vi "(SubVI)AOMvolt-Power Calibration for 1064-v2.vi"(6 "instrument handle":refnum<visa-resource-name>, 7 "error in (no error)":errorcluster {"code" format="%.0x"}) -> (0 "XY Graph":cluster{dbl[], dbl[]}[](graph), 1 "Raw data":T1, 3 "Choosed AOM volt":dbl, 4 "Choosed laser power (mW)":dbl format="%#_13g")   [LabVIEW 2014]
uses:
  <vilib>/Analysis/polynomials.llb/Scalar Polynomial Evaluation (DBL).vi
  <vilib>/Utility/file.llb/Write To Spreadsheet File (DBL).vi
  <vilib>/Analysis/NI_AALPro.lvlib
panel:
  out "Voltage for AOM":dbl
  out "powermeter readout (mW)":dbl
  in  "scan step #":dbl=20.0
  in  "Set laser power (mW)":dbl=10.0 format="%#_13g"
  in  "Scanning cycles":dbl=1.0
  in  "milliseconds to wait":u32=300
  out "voltage step size":dbl=0.25
  in  "Min voltage":dbl=0.1
  in  "Max voltage":dbl=5.0
  in  "save cal curve?":bool
  out "Fit AOM volt(V)":dbl[](array[numeric])
  out "Fit laser power (mW)":dbl[](array[numeric])
  out "Polynomial Coefficients":dbl[](array[numeric]) format="%0.2f"
  out "power":dbl
  out "current voltage":dbl
  in  "stop":bool
  # "continuous scaning power \nover AOM voltage range"
  # "**activate \ncontinuous power\ncontinuous AOM"
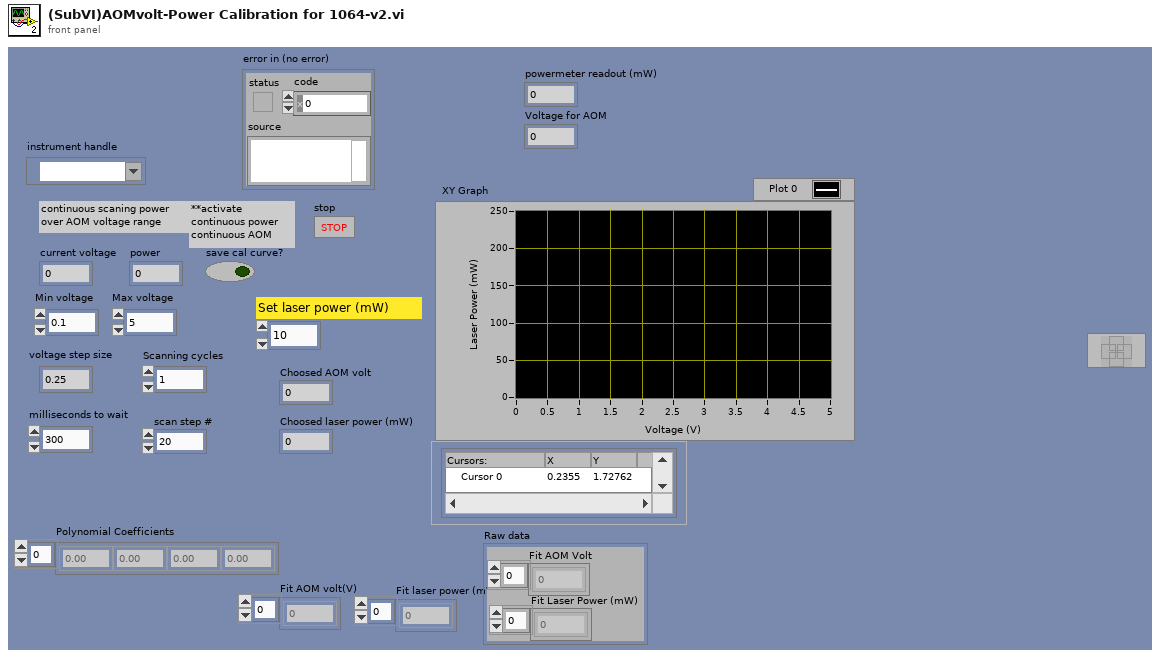
[diagram p1: front panel]
types:
  T1 = cluster{"Fit AOM Volt":dbl[], "Fit Laser Power (mW)":dbl[]}
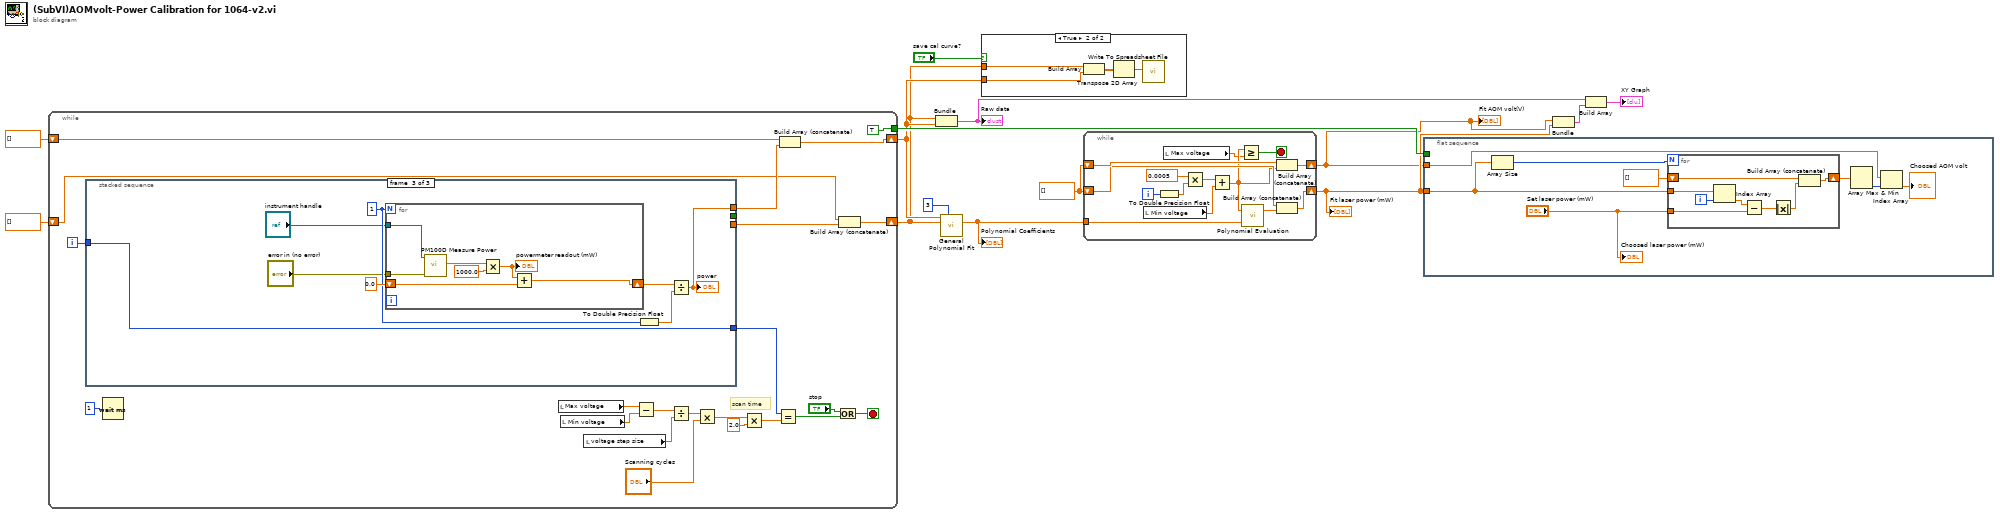
[diagram p0: block diagram]
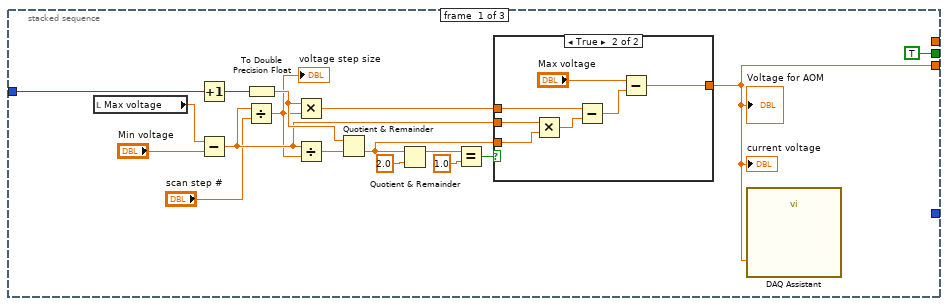
[diagram p3: hidden frame]
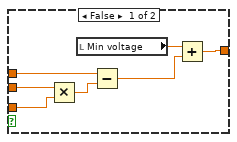
[diagram p4: hidden frame]
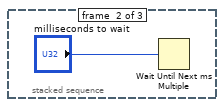
[diagram p5: hidden frame]
diagram:
  w10 = dbl[] []
  n1 = while {
    shift-right: [w34] -> w7
    shift-left: dbl[] [] -> [w31]
    shift-right: [w35] -> w6
    shift-left: dbl[] [] -> [w30]
    tunnel: [TRUE] -> w12
    i -> [w28]
    stop <- w26 stop-if-true
    # "scan time"
    n2 = stacked-sequence {
      tunnel: [w38 _ _] -> w33
      tunnel: [_ _ w72] -> w32
      tunnel: [TRUE _ _] -> _
      tunnel: w28 -> [w45 _ w75]
      tunnel: [_ _ w75] -> w25
      frame #0 {
        n3 = local read "Max voltage"() -> (w43:dbl)
        n4 = Increment(x=w45) -> (x+1=w52:i32)
        n5 = Subtract(x=w43, y="Min voltage") -> (x-y=w41:dbl)
        n6 = Divide(x=w41, y="scan step #") -> (x/y=w39:dbl)
        "voltage step size" <- w39
        n7 = To Double Precision Float(number=w52) -> (double precision float=w44:dbl)
        n8 = Multiply(x=w44, y=w39) -> (x*y=w51:dbl)
        n9 = Divide(x=w41, y=w39) -> (x/y=w42:dbl)
        n10 = Quotient & Remainder(x=w44, y=w42) -> (floor(x/y)=w46:dbl)  [unwired: 1 out]
        n11 = Quotient & Remainder(x=w46, y=2.0) -> (x-y*floor(x/y)=w48:dbl)  [unwired: 1 out]
        n12 = Equal?(x=w48, y=1.0) -> (x = y?=w49:bool)
        n13 = case shown="True" w49 {
          tunnel: w51 -> [w58 w66]
          tunnel: [w60 w67] -> w38
          tunnel: w46 -> [w59 w63]
          tunnel: w41 -> [w55 w61]
          frame False {
            n14 = Multiply(x=w55, y=w59) -> (x*y=w57:dbl)
            n15 = local read "Min voltage"() -> (w54:dbl)
            n16 = Subtract(x=w58, y=w57) -> (x-y=w56:dbl)
            n17 = Add(x=w54, y=w56) -> (x+y=w60:dbl)
          }
          frame True {
            n18 = Multiply(x=w61, y=w63) -> (x*y=w65:dbl)
            n19 = Subtract(x=w66, y=w65) -> (x-y=w64:dbl)
            n20 = Subtract(x="Max voltage", y=w64) -> (x-y=w67:dbl)
          }
        }
        "current voltage" <- w38
        "Voltage for AOM" <- w38
        n21 = call "DAQ Assistant"("data"=w38) -> ()  [unwired: 17 in, 2 out]
      }
      frame #1 {
        n22 = Wait Until Next ms Multiple(millisecond multiple="milliseconds to wait") -> ()  [unwired: 1 out]
      }
      frame #2 {
        w73 = 1
        n23 = for {
          N: w73 -> [_]
          shift-right: [w83] -> w74
          shift-left: 0.0 -> [w82]
          tunnel: "instrument handle" -> [w81]
          tunnel: "error in (no error)" -> [w80]
          n24 = call <instrlib>:"PM100D Measure Power.vi"("error in (no error)"=w80, "instrument handle"=w81) -> ("Power"=w79:dbl)  [unwired: 7 in, 2 out]
          n25 = Multiply(x=w79, y=1000.0) -> (x*y=w77:dbl)
          "powermeter readout (mW)" <- w77
          n26 = Add(x=w77, y=w82) -> (x+y=w83:dbl)
        }
        n27 = To Double Precision Float(number=w73) -> (double precision float=w71:dbl)
        n28 = Divide(x=w74, y=w71) -> (x/y=w72:dbl)
        "power" <- w72
      }
    }
    n29 = Wait (ms)(milliseconds to wait=u32 1) -> ()  [unwired: 1 out]
    n30 = local read "Max voltage"() -> (w23:dbl)
    n31 = local read "Min voltage"() -> (w22:dbl)
    n32 = local read "voltage step size"() -> (w20:dbl)
    n33 = Subtract(x=w23, y=w22) -> (x-y=w21:dbl)
    n34 = Divide(x=w21, y=w20) -> (x/y=w19:dbl)
    n35 = Multiply(x=w19, y="Scanning cycles") -> (x*y=w16:dbl)
    n36 = Multiply(x=w16, y=2.0) -> (x*y=w17:dbl)
    n37 = Equal?(x=w25, y=w17) -> (x = y?=w24:bool)
    n38 = Build Array (concatenate)(w31, w32) -> (w34:dbl[])
    n39 = Or(x="stop", y=w24) -> (x .or. y?=w26:bool)
    n40 = Build Array (concatenate)(w30, w33) -> (w35:dbl[])
  }
  n41 = Bundle(w6, w7) -> (w1:cluster{dbl[], dbl[]})  [unwired: 1 out]
  "Raw data" <- w1
  n42 = call <vilib>:"General Polynomial Fit.vi"("Y"=w7, "polynomial order"=3, "X"=w6) -> ("Polynomial Coefficients"=w4:dbl[])  [unwired: 9 in, 3 out]
  "Polynomial Coefficients" <- w4
  n43 = case shown="True" "save cal curve?" {
    tunnel: w7 -> [_ w87]
    tunnel: w6 -> [_ w86]
    frame False {
    }
    frame True {
      n44 = Build Array(w86, w87) -> (w85:dbl[][])
      n45 = Transpose 2D Array(2D array=w85) -> (transposed array=w84:dbl[][])
      n46 = call-poly <vilib>:"Write To Spreadsheet File.vi"("2D data"=w84) -> ()  [unwired: 5 in, 3 out]
    }
  }
  n47 = while {
    tunnel: w4 -> [w97]
    shift-right: [w96] -> w2
    shift-left: w10 -> [w93]
    shift-right: [w94] -> w3
    shift-left: w10 -> [w92]
    i -> [w101]
    stop <- w90 stop-if-true
    n48 = local read "Min voltage"() -> (w88:dbl)
    n49 = To Double Precision Float(number=w101) -> (double precision float=w100:dbl)
    n50 = local read "Max voltage"() -> (w89:dbl)
    n51 = Multiply(x=0.0005, y=w100) -> (x*y=w98:dbl)
    n52 = Add(x=w98, y=w88) -> (x+y=w91:dbl)
    n53 = Greater Or Equal?(x=w91, y=w89) -> (x >= y?=w90:bool)
    n54 = call-poly <vilib>:"Polynomial Evaluation.vi"("P(x)"=w97, "a"=w91) -> ("P(a)"=w95:dbl)  [unwired: 1 out]
    n55 = Build Array (concatenate)(w93, w91) -> (w96:dbl[])
    n56 = Build Array (concatenate)(w92, w95) -> (w94:dbl[])
  }
  "Fit laser power (mW)" <- w3
  "Fit AOM volt(V)" <- w2
  n57 = flat-sequence {
    tunnel: w12 -> [_]
    tunnel: w3 -> [w103]
    tunnel: w2 -> [w106]
    frame #0 {
      n58 = Array Size(array=w103) -> (size(s)=w102:i32)
      n59 = for {
        N: w102 -> [_]
        tunnel: w103 -> [w117]
        tunnel: "Set laser power (mW)" -> [w114]
        shift-right: [w111] -> w107
        shift-left: dbl[] [] -> [w110]
        i -> [w116]
        n60 = Index Array(array=w117, index=w116) -> (element=w115:dbl)
        n61 = Subtract(x=w115, y=w114) -> (x-y=w113:dbl)
        n62 = Absolute Value(x=w113) -> (abs(x)=w112:dbl)
        n63 = Build Array (concatenate)(w110, w112) -> (w111:dbl[])
      }
      n64 = Array Max & Min(array=w107) -> (min index (indices)=w105:i32)  [unwired: 3 out]
      n65 = Index Array(array=w106, index=w105) -> (element=→"Choosed AOM volt":dbl)
      "Choosed laser power (mW)" <- "Set laser power (mW)"
    }
  }
  n66 = Bundle(w2, w3) -> (w9:cluster{dbl[], dbl[]})  [unwired: 1 out]
  n67 = Build Array(w1, w9) -> (→"XY Graph":cluster{dbl[], dbl[]}[])
